vi "Results_Row_Per_Channel.vi"(0 "Duplicate Channel":bool, 1 "Duplicate Metadata channels":string[](array[string]), 2 "Analysis_info_cluster":T2={"Colour"=0, "Inst type"=enum."Pitot-static tube", "Inst name"="Manometer voltage", "Symbol"="U", "Code name"="", "Extra Info"="U", "Inst Array"=enum."PWA", "U"=0.0, "u^2"=0.0, "u^3"=0.0, "u^4"=0.0, "Skew_u"=0.0, "Kurt_u"=0.0, "Sd Error in Mean"=0.0, "% u'/U"=0.0, "X"=0.0, "Y"=0.0, "Z"=0.0, "Timescale integral Estimate"=0.0, "Sd Error in Variance"=0.0, "Calib File"=path "", "Calib Constants"=[], "Output Position"=FALSE, "Stats"=enum."None", "Av Sampling Rate"=0.0, "Av No of Samples"=0.0, "Total Meas Time (s)"=0.0, "OrigChName"="", "Max value"=0.0, "Min value"=0.0, "Req Sample Rate Hz"=0.0, "Sync Delay Time (s)"=0.0, "Ch No"=0, "Device"="", "Use Latest Calib"=FALSE, "Port"="", "Metadata Ch Names"=[], "Metadata Ch Values"=[], "Label"="", "chState"=enum."Solo", "Point Drift"=0.0, "inputConfig"=""} {"Kurt_u" format="%_3g"; "u^4" format="%_3g"; "u^3" format="%_3g"; "Sd Error in Variance" format="%_3g"; "u^2" format="%_3g"; "Sd Error in Mean" format="%_3g"; "U" format="%_3g"; "Sync Delay Time (s)" format="%.4f"; "Total Meas Time (s)" format="%_5g"; "Skew_u" format="%_3g"; "% u'/U" format="%_3g"}, 3 "Histogram Info":T1 {"X array" format="%^_5g"; "Y array" format="%^_5g"}, 4 "Index":i32) -> (5 "Channel Names":string[](array[string]), 6 "Channel Values":string[](array[string]))   [LabVIEW 2022 SP3]
uses:
  Acquisition/PWA/PWAtasksGLOBAL.vi
  Controls/Post_Process.ctl
  Globals/Meas_global.vi
  Controls/Inst_type.ctl
  FFID/FFID Calib Constants index.ctl
  Controls/Instrument_Array.ctl
  Controls/Analysis_info_cluster.ctl
  Controls/XY_Plot_Cluster.ctl
  Controls/channelState.ctl
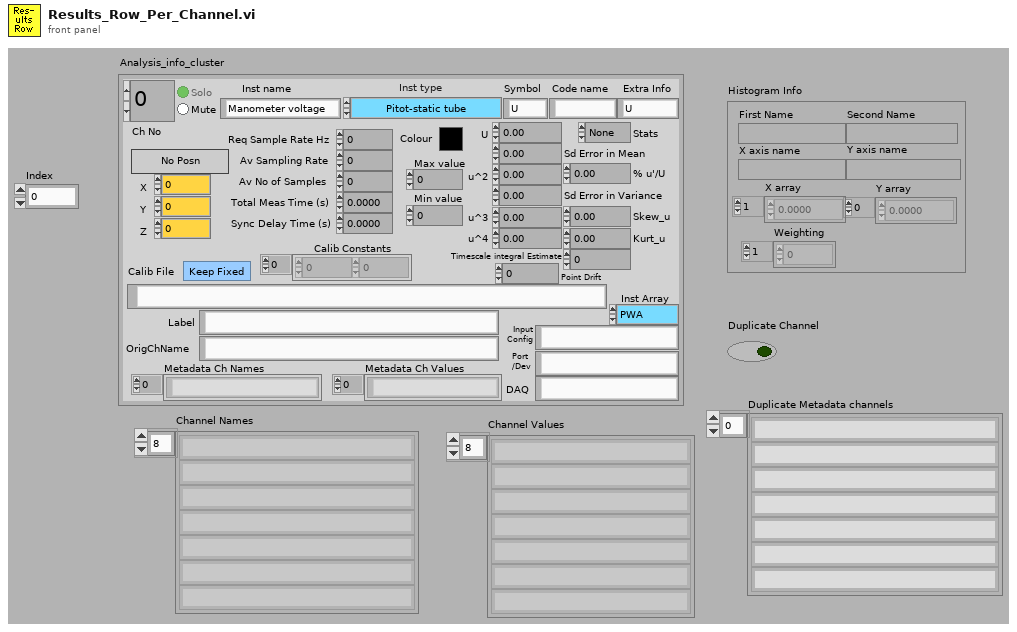
[diagram p1: front panel]
types:
  T1 = typedef "XY_Plot_Cluster.ctl" = cluster{"First Name":string, "Second Name":string, "X axis name":string, "Y axis name":string, "X array":dbl[], "Y array":dbl[], "Weighting":dbl[]}
  T2 = typedef "Analysis_info_cluster.ctl" = cluster{"Colour":u32, "Inst type":T3, "Inst name":string, "Symbol":string, "Code name":string, "Extra Info":string, "Inst Array":T4, "U":dbl, "u^2":dbl, "u^3":dbl, "u^4":dbl, "Skew_u":dbl, "Kurt_u":dbl, "Sd Error in Mean":dbl, "% u'/U":dbl, "X":dbl, "Y":dbl, "Z":dbl, "Timescale integral Estimate":dbl, "Sd Error in Variance":dbl, "Calib File":path, "Calib Constants":dbl[], "Output Position":bool, "Stats":enum16{"None", "Basic", "Full"}, "Av Sampling Rate":dbl, "Av No of Samples":dbl, "Total Meas Time (s)":dbl, "OrigChName":string, "Max value":dbl, "Min value":dbl, "Req Sample Rate Hz":dbl, "Sync Delay Time (s)":dbl, "Ch No":i16, "Device":string, "Use Latest Calib":bool, "Port":string, "Metadata Ch Names":string[], "Metadata Ch Values":string[], "Label":string, "chState":T5, "Point Drift":dbl, "inputConfig":string}
  T3 = typedef "Inst_type.ctl" = enum16{"Raw voltage", "Raw with zero offsetting", "Propeller anemometer", "Pressure Transducer", "Pitot-static tube", "Hot wire", "Cross wire 1", "Cross wire 2", "Generic Linear", "Generic Polynomial", "Generic BackPoly", "Fast FID", "Thermocouple", "Cold wire", "Pulsed Wire", "LDA Vel", "LDA Tran time", "LDA Arr time", "Microphone"}
  T4 = typedef "Instrument_Array.ctl" = enum16{"PWA", "LDA", "Analogue"}
  T5 = typedef "channelState.ctl" = enum32{"No Selection", "Solo", "Mute"}
  T6 = enum16{"Mean only", "2nd Order Stats", "4th Order Stats"}
  T7 = typedef "Post_Process.ctl" = enum16{"Take New Data", "Post Process Raw Data File"}
  T8 = typedef "FFID Calib Constants index.ctl" = u16
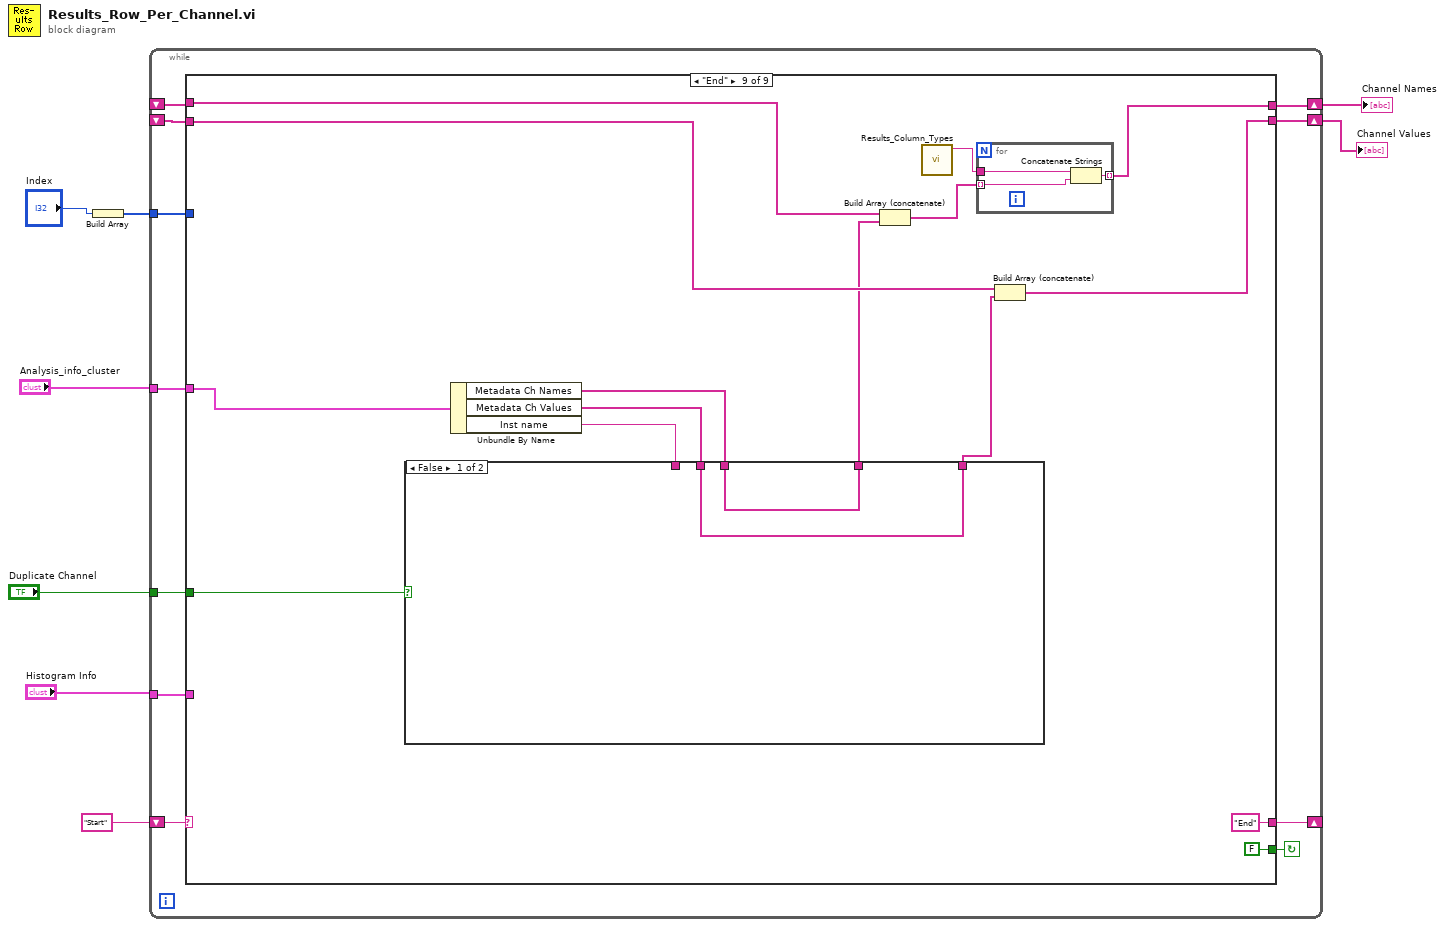
[diagram p0: block diagram]
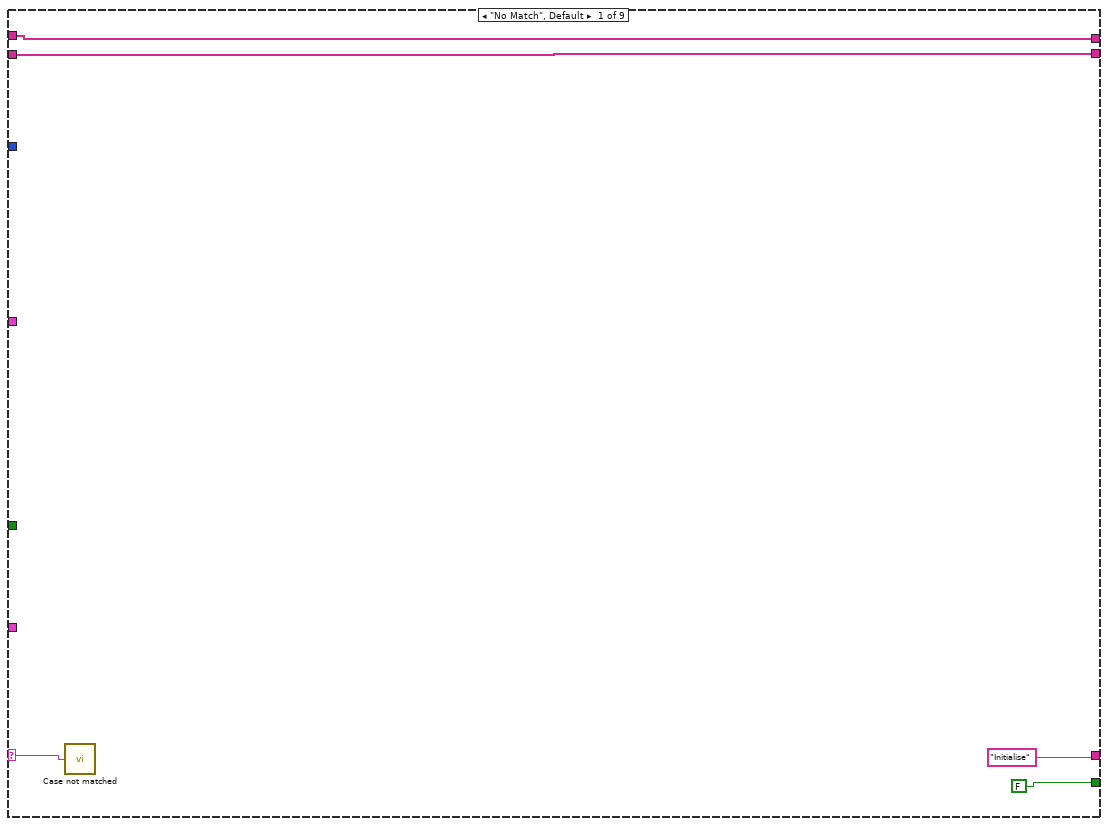
[diagram p2: hidden frame]
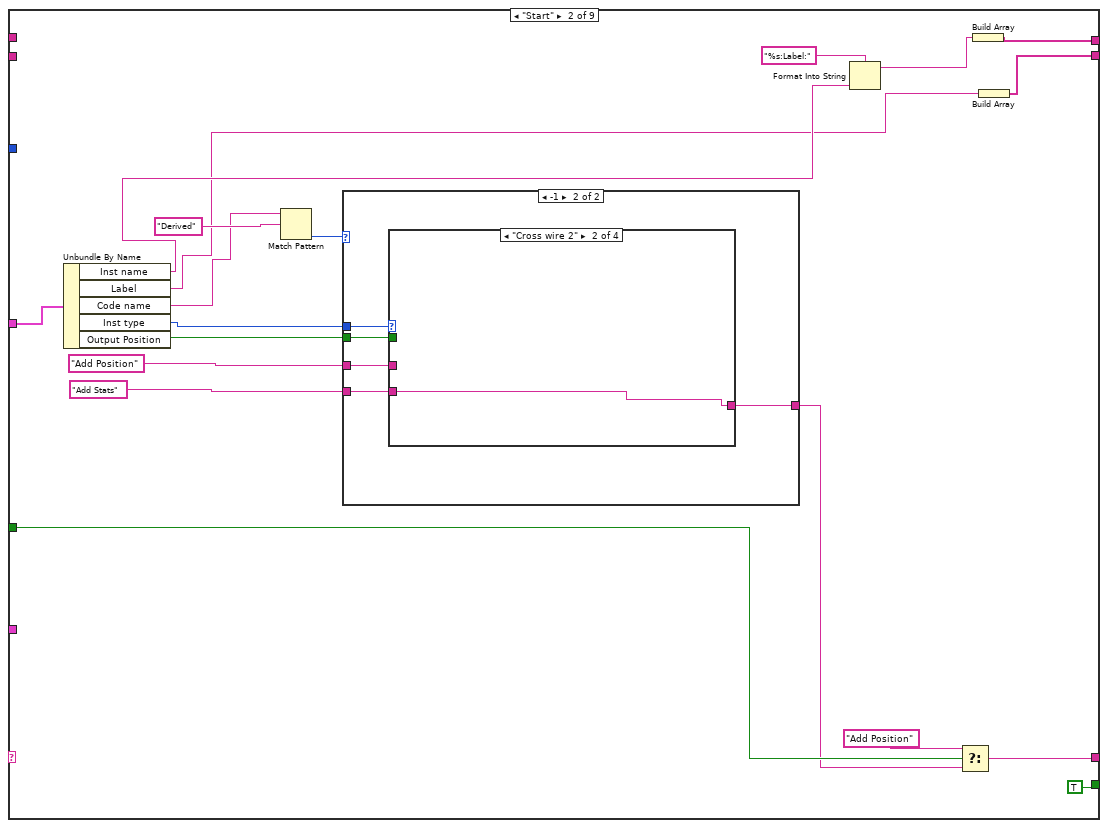
[diagram p3: hidden frame]
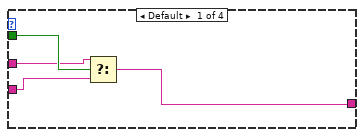
[diagram p5: hidden frame]
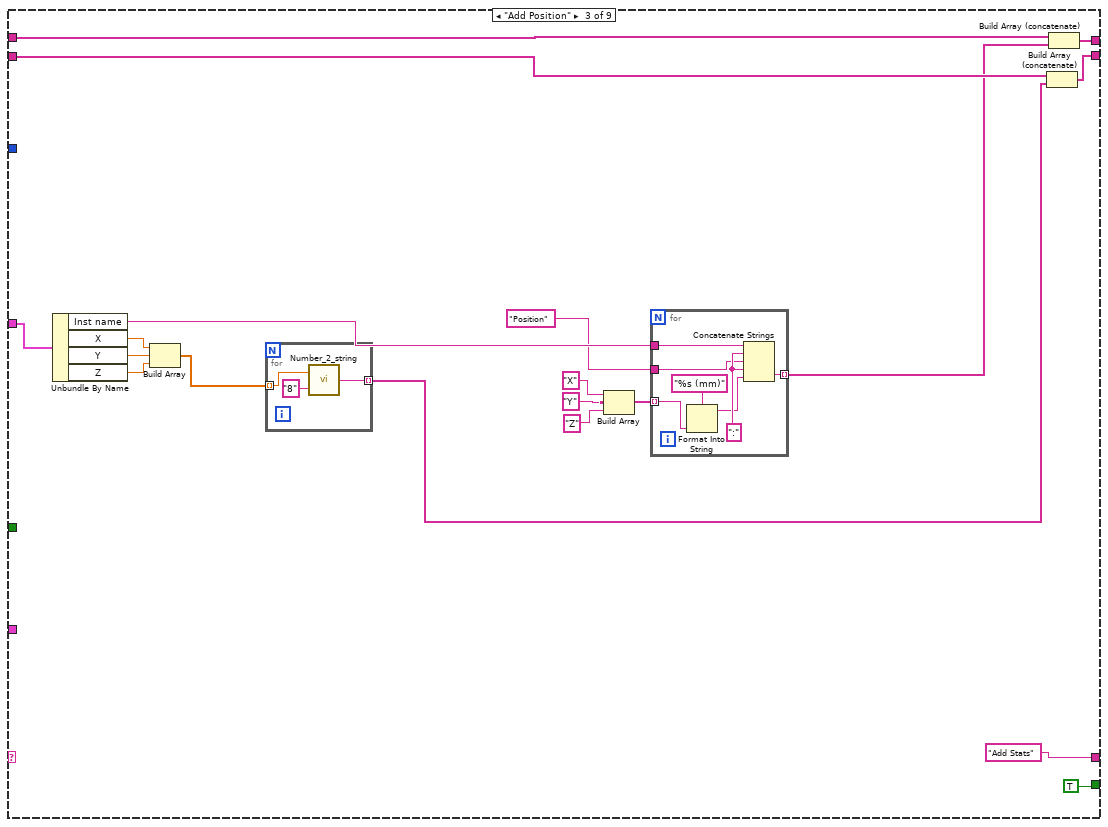
[diagram p8: hidden frame]
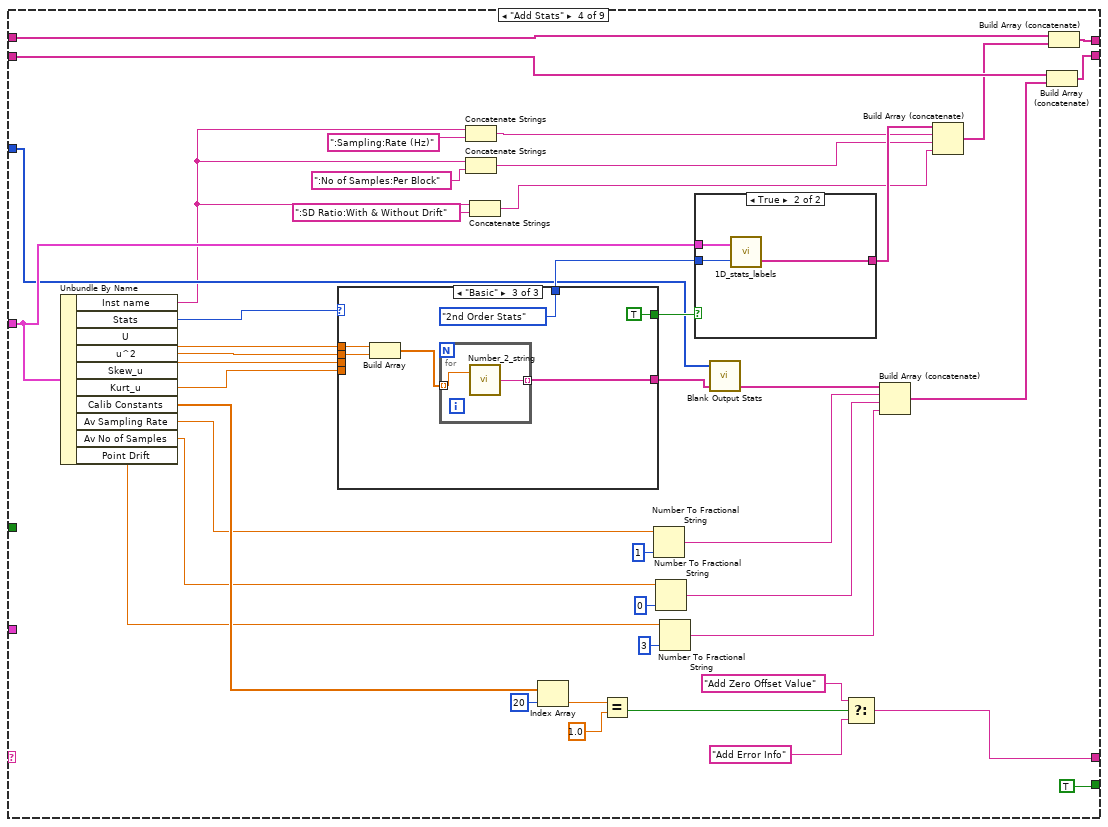
[diagram p9: hidden frame]
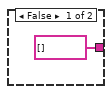
[diagram p10: hidden frame]
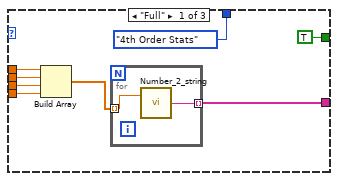
[diagram p11: hidden frame]
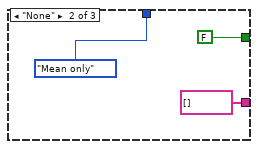
[diagram p12: hidden frame]
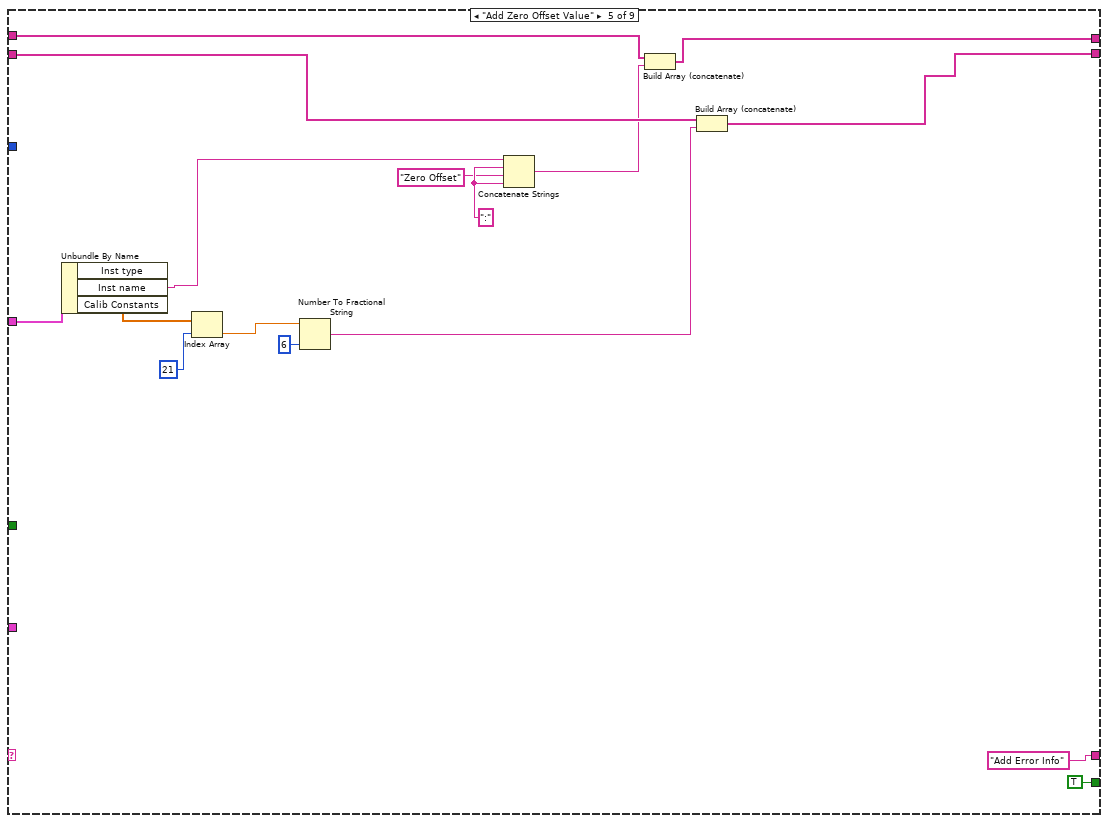
[diagram p13: hidden frame]
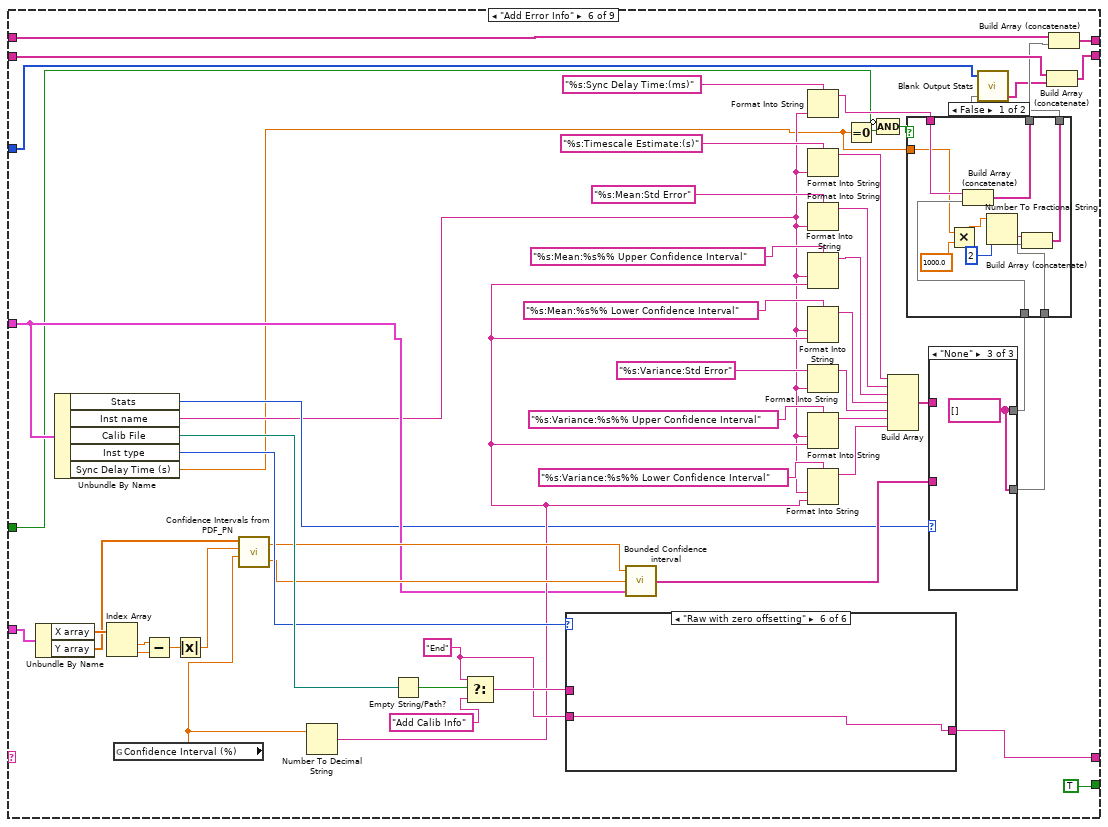
[diagram p14: hidden frame]
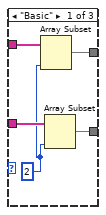
[diagram p16: hidden frame]
diagram:
  n1 = Build Array("Index") -> (w1:i32[])
  n2 = while {
    shift-left: "Start" -> [w17]
    shift-right: [w18] -> _
    shift-right: [w12] -> w5
    shift-left: _ -> [w13]
    shift-right: [w15] -> w6
    shift-left: _ -> [w14]
    tunnel: "Analysis_info_cluster" -> [w16]
    tunnel: "Histogram Info" -> [w11]
    tunnel: "Duplicate Channel" -> [w10]
    tunnel: w1 -> [w9]
    stop <- w19 continue-if-true
    n3 = case shown="\"End\"" w17 {
      selector: w17 -> [w20 _ _ _ _ _ _ _ _]
      tunnel: [FALSE TRUE TRUE TRUE TRUE TRUE TRUE TRUE FALSE] -> w19
      tunnel: ["Initialise" w31 "Add Stats" w110 "Add Error Info" w214 w255 "End" "End"] -> w18
      tunnel: w16 -> [_ w42 w73 w120 w169 w200 w268 w388 w423]
      tunnel: [w21 w25 w66 w125 w161 w222 w264 w365 w420] -> w15
      tunnel: w14 -> [w21 _ w65 w124 w163 w221 w266 w390 w421]
      tunnel: w13 -> [w22 _ w64 w123 w164 w220 w262 w389 w422]
      tunnel: [w22 w27 w63 w122 w157 w219 w260 w364 w412] -> w12
      tunnel: w11 -> [_ _ _ _ _ w211 _ _ _]
      tunnel: w10 -> [_ w34 _ _ _ w173 _ _ w415]
      tunnel: w9 -> [_ _ _ w106 _ w172 _ _ _]
      frame "No Match", Default {
        n4 = call "Case not matched.vi"("Case Name not Matched"=w20) -> ()
      }
      frame "Start" {
        n5 = Unbundle By Name(w42) -> ("Inst name"=w29:string, "Label"=w26:string, "Code name"=w37:string, "Inst type"=w41:T3, "Output Position"=w35:bool)
        n6 = Match Pattern(string=w37, regular expression="Derived") -> (offset past match=w36:i32)  [unwired: 1 in, 3 out]
        n7 = case shown="-1" w36 {
          tunnel: w41 -> [_ w49]
          tunnel: [w44 w48] -> w32
          tunnel: "Add Position" -> [_ w47]
          tunnel: "Add Stats" -> [w44 w46]
          tunnel: w35 -> [_ w45]
          frame 0, Default {
          }
          frame -1 {
            n8 = case shown="\"Cross wire 2\"" w49 {
              tunnel: [w50 w54 w55 w56] -> w48
              tunnel: w47 -> [w52 _ _ _]
              tunnel: w46 -> [w51 w54 w55 w56]
              tunnel: w45 -> [w53 _ _ _]
              frame Default {
                n9 = Select(t=w52, s=w53, f=w51) -> (s? t:f=w50:string)
              }
              frame "Cross wire 2" {
              }
              frame "LDA Tran time" {
              }
              frame "LDA Arr time" {
              }
            }
          }
        }
        n10 = Format Into String(format string="%s:Label:" ("Format String"), w29) -> (resulting string=w28:string)  [unwired: 2 in, 1 out]
        n11 = Select(t="Add Position", s=w34, f=w32) -> (s? t:f=w31:string)
        n12 = Build Array(w28) -> (w27:string[])
        n13 = Build Array(w26) -> (w25:string[])
      }
      frame "Add Position" {
        n14 = Unbundle By Name(w73) -> ("Inst name"=w72:string, "X"=w71:dbl, "Y"=w70:dbl, "Z"=w69:dbl)
        n15 = Build Array(w71, w70, w69) -> (w68:dbl[])
        n16 = for {
          tunnel: w68 -> [w78] mode=indexing
          tunnel: [w77] -> w67 mode=indexing
          n17 = call "Number_2_string.vi"("precision"="8", "number"=w78) -> ("String"=w77:string)
        }
        n18 = Build Array("X", "Y", "Z") -> (w61:string[])
        n19 = for {
          tunnel: w61 -> [w82] mode=indexing
          tunnel: w72 -> [w85]
          tunnel: [w83] -> w62 mode=indexing
          tunnel: "Position" -> [w79]
          w84 = ":" ("Substring")
          n20 = Format Into String(format string="%s (mm)", w82) -> (resulting string=w80:string)  [unwired: 2 in, 1 out]
          n21 = Concatenate Strings(w85, w84, w79, w84, w80) -> (w83:string)
        }
        n22 = Build Array (concatenate)(w65, w67) -> (w66:string[])
        n23 = Build Array (concatenate)(w64, w62) -> (w63:string[])
      }
      frame "Add Stats" {
        n24 = Unbundle By Name(w120) -> ("Inst name"=w92:string, "Stats"=w117:enum16{"None", "Basic", "Full"}, "U"=w128:dbl, "u^2"=w127:dbl, "Skew_u"=w126:dbl, "Kurt_u"=w121:dbl, "Calib Constants"=w113:dbl[], "Av Sampling Rate"=w99:dbl, "Av No of Samples"=w97:dbl, "Point Drift"=w87:dbl)
        n25 = case shown="\"Basic\"" w117 {
          tunnel: w128 -> [w140 _ w151]
          tunnel: w127 -> [w139 _ w150]
          tunnel: w126 -> [w138 _ _]
          tunnel: [w136 string[] [] w148] -> w107
          tunnel: w121 -> [w135 _ _]
          tunnel: [T6."4th Order Stats" ("Mode selector") T6."Mean only" ("Mode selector") T6."2nd Order Stats" ("Mode selector")] -> w118
          tunnel: [TRUE FALSE TRUE] -> w108
          frame "Full" {
            n26 = Build Array(w140, w139, w138, w135) -> (w137:dbl[])
            n27 = for {
              tunnel: w137 -> [w142] mode=indexing
              tunnel: [w141] -> w136 mode=indexing
              n28 = call "Number_2_string.vi"("number"=w142) -> ("String"=w141:string)  [unwired: 1 in]
            }
          }
          frame "None" {
          }
          frame "Basic" {
            n29 = Build Array(w151, w150) -> (w149:dbl[])
            n30 = for {
              tunnel: w149 -> [w153] mode=indexing
              tunnel: [w152] -> w148 mode=indexing
              n31 = call "Number_2_string.vi"("number"=w153) -> ("String"=w152:string)  [unwired: 1 in]
            }
          }
        }
        n32 = Concatenate Strings(w92, ":Sampling:Rate (Hz)" ("string")) -> (w101:string)
        n33 = Concatenate Strings(w92, ":No of Samples:Per Block") -> (w100:string)
        n34 = Concatenate Strings(w92, ":SD Ratio:With & Without Drift" ("string")) -> (w90:string)
        n35 = Index Array(array=w113, index=20) -> (element=w116:dbl)
        n36 = Equal?(x=w116, y=1.0) -> (x = y?=w112:bool)
        n37 = Number To Fractional String(number=w99, precision (6)=i16 1) -> (F-format string=w95:string)  [unwired: 2 in]
        n38 = Number To Fractional String(number=w97, precision (6)=i16 0) -> (F-format string=w94:string)  [unwired: 2 in]
        n39 = Number To Fractional String(number=w87, precision (6)=i16 3) -> (F-format string=w86:string)  [unwired: 2 in]
        n40 = case shown="True" w108 {
          tunnel: w120 -> [_ w132]
          tunnel: [string[] [] ("Output") w131] -> w102
          tunnel: w118 -> [_ w130]
          frame False {
          }
          frame True {
            n41 = call "1D_stats_labels.vi"("Mode selector"=w130, "Analysis Info Cluster"=w132) -> ("Output"=w131:string[])  [unwired: 1 in]
          }
        }
        n42 = call "Blank Output Stats.vi"("Ch Values in"=w107, "Indices"=w106) -> ("Ch Values Out"=w96:string[])  [unwired: 2 in, 1 out]
        n43 = Select(t="Add Zero Offset Value", s=w112, f="Add Error Info") -> (s? t:f=w110:string)
        n44 = Build Array (concatenate)(w96, w95, w94, w86) -> (w93:string[])
        n45 = Build Array (concatenate)(w102, w101, w100, w90) -> (w103:string[])
        n46 = Build Array (concatenate)(w124, w93) -> (w125:string[])
        n47 = Build Array (concatenate)(w123, w103) -> (w122:string[])
      }
      frame "Add Zero Offset Value" {
        w160 = ":" ("Substring")
        n48 = Unbundle By Name(w169) -> ("Inst name"=w159:string, "Calib Constants"=w168:dbl[])  [unwired: 1 out]
        n49 = Index Array(array=w168, index=21) -> (element=w165:dbl)
        n50 = Number To Fractional String(number=w165, precision (6)=i16 6) -> (F-format string=w162:string)  [unwired: 2 out]
        n51 = Concatenate Strings(w159, w160, "Zero Offset" ("string"), w160) -> (w158:string)
        n52 = Build Array (concatenate)(w164, w158) -> (w157:string[])
        n53 = Build Array (concatenate)(w163, w162) -> (w161:string[])
      }
      frame "Add Error Info" {
        w212 = "End"
        n54 = Unbundle By Name(w211) -> ("X array"=w206:dbl[], "Y array"=w205:dbl[])
        n55 = Unbundle By Name(w200) -> ("Stats"=w183:enum16{"None", "Basic", "Full"}, "Inst name"=w181:string, "Calib File"=w218:path, "Inst type"=w213:T3, "Sync Delay Time (s)"=w176:dbl)
        n56 = Index Array(array=w206) -> (element #1=w207:dbl, element #2=w208:dbl)  [unwired: 2 in]
        n57 = global read "Meas_global.vi" "Confidence Interval (%)"() -> (w202:dbl)
        n58 = Subtract(x=w207, y=w208) -> (x-y=w209:dbl)
        n59 = Absolute Value(x=w209) -> (abs(x)=w210:dbl)
        n60 = call "Confidence Intervals from PDF_PN.vi"("Desired confidence interval (%)"=w202, "PDF bin width"=w210, "Marginal 1D PDF"=w205) -> ("Lower limit scale factor on SD or SE"=w203:dbl, "Upper limit scale factor on SD or SE"=w204:dbl)  [unwired: 1 in]
        n61 = Number To Decimal String(number=w202) -> (decimal integer string=w201:string)  [unwired: 1 in]
        n62 = Empty String/Path?(string/path=w218) -> (empty?=w217:bool)
        n63 = Select(t=w212, s=w217, f="Add Calib Info") -> (s? t:f=w215:string)
        n64 = case shown="\"Raw with zero offsetting\"" w213 {
          tunnel: [w244 w245 w246 w247 w248 w249] -> w214
          tunnel: w215 -> [w244 _ _ _ _ _]
          tunnel: w212 -> [_ w245 w246 w247 w248 w249]
          frame "Propeller anemometer", Default {
          }
          frame "Cross wire 2" {
          }
          frame "LDA Tran time" {
          }
          frame "LDA Arr time" {
          }
          frame "Raw voltage" {
          }
          frame "Raw with zero offsetting" {
          }
        }
        n65 = call "Bounded Confidence interval.vi"("Analysis_info_cluster"=w200, "Lower limit scale factor on SD or SE"=w203, "Upper limit scale factor on SD or SE"=w204) -> ("Error values"=w184:string[])
        n66 = Format Into String(format string="%s:Sync Delay Time:(ms)", w181) -> (resulting string=w180:string)  [unwired: 2 in, 1 out]
        n67 = Format Into String(format string="%s:Timescale Estimate:(s)", w181) -> (resulting string=w192:string)  [unwired: 2 in, 1 out]
        n68 = Format Into String(format string="%s:Mean:Std Error", w181) -> (resulting string=w191:string)  [unwired: 2 in, 1 out]
        n69 = Format Into String(format string="%s:Mean:%s%% Upper Confidence Interval", w181, w201) -> (resulting string=w190:string)  [unwired: 2 in, 1 out]
        n70 = Format Into String(format string="%s:Mean:%s%% Lower Confidence Interval", w181, w201) -> (resulting string=w189:string)  [unwired: 2 in, 1 out]
        n71 = Format Into String(format string="%s:Variance:Std Error", w181) -> (resulting string=w188:string)  [unwired: 2 in, 1 out]
        n72 = Format Into String(format string="%s:Variance:%s%% Upper Confidence Interval", w181, w201) -> (resulting string=w187:string)  [unwired: 2 in, 1 out]
        n73 = Format Into String(format string="%s:Variance:%s%% Lower Confidence Interval", w181, w201) -> (resulting string=w186:string)  [unwired: 2 in, 1 out]
        n74 = Equal To 0?(x=w176) -> (x = 0?=w175:bool)
        n75 = Compound Arithmetic op=AND(invert w173, w175) -> (w174:bool)
        n76 = Build Array(w192, w191, w190, w189, w188, w187, w186) -> (w185:string[])
        n77 = case shown="\"None\"" w183 {
          tunnel: w185 -> [w240 w242 _]
          tunnel: [w239 w242 w243] -> w179
          tunnel: w184 -> [w238 w241 _]
          tunnel: [w237 w241 w243] -> w177
          frame "Basic" {
            w236 = 2 ("length")
            n78 = Array Subset(array=w240, length=w236) -> (w239:string[])  [unwired: 1 in]
            n79 = Array Subset(array=w238, length=w236) -> (w237:string[])  [unwired: 1 in]
          }
          frame "Full" {
          }
          frame "None" {
            w243 = string[] []
          }
        }
        n80 = case shown="False" w174 {
          tunnel: w180 -> [w233 _]
          tunnel: w179 -> [w232 w235]
          tunnel: [w231 w235] -> w178
          tunnel: w177 -> [w230 w234]
          tunnel: [w229 w234] -> w171
          tunnel: w176 -> [w228 _]
          frame False {
            n81 = Multiply(x=w228, y=1000.0) -> (x*y=w226:dbl)
            n82 = Build Array (concatenate)(w233, w232) -> (w231:string[])
            n83 = Number To Fractional String(number=w226, precision (6)=i16 2) -> (F-format string=w225:string)  [unwired: 2 in]
            n84 = Build Array (concatenate)(w225, w230) -> (w229:string[])
          }
          frame True {
          }
        }
        n85 = call "Blank Output Stats.vi"("Ch Values in"=w171, "Indices"=w172) -> ("Ch Values Out"=w170:string[])  [unwired: 2 in, 1 out]
        n86 = Build Array (concatenate)(w221, w170) -> (w222:string[])
        n87 = Build Array (concatenate)(w220, w178) -> (w219:string[])
      }
      frame "Add Calib Info" {
        w250 = T8 19 items=["0 Coeff A", "1 Coeff B", "2 Coeff C", "3 FFID Bkgnd", "4 FFID Bkgnd Variance", "5 FFID Bkgnd Volts", "6 FFID Bkgnd Time", "7 GMU Source ppm/%density", "8 Orig Bkgnd Time", "9 Orig Bknd volts", "10 Orig bkgnd Variance", "11 Intermittency Theshold", "12 Intermittency", "13 Head Temp", "14 Exhaust Temp", "15", "16", "17", "18 Calibration Drift %", "19 Calibration Interval Minutes"] ("FFID")
        w251 = T8 18 items=["0 Coeff A", "1 Coeff B", "2 Coeff C", "3 FFID Bkgnd", "4 FFID Bkgnd Variance", "5 FFID Bkgnd Volts", "6 FFID Bkgnd Time", "7 GMU Source ppm/%density", "8 Orig Bkgnd Time", "9 Orig Bknd volts", "10 Orig bkgnd Variance", "11 Intermittency Theshold", "12 Intermittency", "13 Head Temp", "14 Exhaust Temp", "15", "16", "17", "18 Calibration Drift %", "19 Calibration Interval Minutes"] ("FFID")
        n88 = Unbundle By Name(w268) -> ("Inst name"=w259:string, "Inst type"=w258:T3, "Calib Constants"=w252:dbl[], "Calib File"=w267:path)
        n89 = Format Into String(format string="%s:Calibration:Filename" ("Format String"), w259) -> (resulting string=w261:string)  [unwired: 2 in, 1 out]
        n90 = Strip Path(path=w267) -> (name=w265:string)  [unwired: 1 out]
        n91 = case shown="\"Generic Linear\", Default" w258 {
          tunnel: [w275 w280 w297 w303 w310 w333] -> w264
          tunnel: w266 -> [w273 w281 w298 w304 w311 w334]
          tunnel: w265 -> [w274 w279 w296 w302 _ w327]
          tunnel: w252 -> [_ _ w289 _ _ w326]
          tunnel: w262 -> [w272 w278 w295 w301 w307 w321]
          tunnel: w261 -> [w270 w277 w294 w299 w305 w320]
          tunnel: [w271 w276 w293 w300 w306 w315] -> w260
          tunnel: w259 -> [_ _ w291 _ _ w314]
          tunnel: w250 -> [_ _ _ _ _ w313]
          tunnel: w251 -> [_ _ _ _ _ w312]
          frame "Propeller anemometer" {
            n92 = Build Array (concatenate)(w272, w270) -> (w271:string[])
            n93 = Build Array (concatenate)(w273, w274) -> (w275:string[])
          }
          frame "Pressure Transducer" {
            n94 = Build Array (concatenate)(w278, w277) -> (w276:string[])
            n95 = Build Array (concatenate)(w281, w279) -> (w280:string[])
          }
          frame "Cold wire" {
            n96 = Index Array(array=w289, index #1=7 ("index"), index #2=6 ("index")) -> (element #1=w283:dbl, element #2=w282:dbl)
            n97 = Format Into String(format string="%s:Mean:Voltage" ("Format String"), w291) -> (resulting string=w290:string)  [unwired: 2 in, 1 out]
            n98 = Divide(x=w283, y=w282) -> (x/y=w287:dbl)
            n99 = Number To Fractional String(number=w287, precision (6)=i16 6) -> (F-format string=w285:string)  [unwired: 2 in]
            n100 = Build Array (concatenate)(w295, w294, w290) -> (w293:string[])
            n101 = Build Array (concatenate)(w298, w296, w285) -> (w297:string[])
          }
          frame "Pitot-static tube" {
            n102 = Build Array (concatenate)(w301, w299) -> (w300:string[])
            n103 = Build Array (concatenate)(w304, w302) -> (w303:string[])
          }
          frame "Pulsed Wire" {
            n104 = global read "PWAtasksGLOBAL.vi" "PWA Calib. File Path"() -> (w309:path)
            n105 = Strip Path(path=w309) -> (name=w308:string)  [unwired: 1 out]
            n106 = Build Array (concatenate)(w307, w305) -> (w306:string[])
            n107 = Build Array (concatenate)(w311, w308) -> (w310:string[])
          }
          frame "Generic Linear", Default {
            n108 = global read "Meas_global.vi" "Post Process"() -> (w329:T7)
            n109 = Index Array(array=w326, index=w312) -> (element=w332:dbl)
            n110 = Format Into String(format string="%s:Calibration:Drift:%%" ("Format String"), w314) -> (resulting string=w317:string)  [unwired: 2 in, 1 out]
            n111 = Not A Number/Path/Refnum?(number/path/refnum=w332) -> (NaN/Path/Refnum?=w331:bool)
            n112 = Equal?(x=w329, y=Post_Process."Post Process Raw Data File" ("Post Process")) -> (x = y?=w322:bool)
            n113 = case shown="False" w331 {
              tunnel: [w344 w349] -> w328
              tunnel: w332 -> [w345 _]
              tunnel: w322 -> [_ w351]
              tunnel: w327 -> [_ w348]
              frame False {
                n114 = Number To Fractional String(number=w345, precision (6)=i16 2) -> (F-format string=w344:string)  [unwired: 2 out]
              }
              frame True {
                n115 = Concatenate Strings(w348, "_Drift_Place_Holder" ("Substring")) -> (w350:string)
                n116 = Select(t="No Info", s=w351, f=w350) -> (s? t:f=w349:string)
              }
            }
            n117 = Index Array(array=w326, index=w313) -> (element=w325:dbl)
            n118 = Not A Number/Path/Refnum?(number/path/refnum=w325) -> (NaN/Path/Refnum?=w324:bool)
            n119 = case shown="False" w324 {
              tunnel: [w335 w340] -> w323
              tunnel: w325 -> [w336 _]
              tunnel: w322 -> [_ w342]
              tunnel: w327 -> [_ w339]
              frame False {
                n120 = Number To Fractional String(number=w336, precision (6)=i16 2) -> (F-format string=w335:string)  [unwired: 2 out]
              }
              frame True {
                n121 = Concatenate Strings(w339, "_Interval_Place_Holder" ("Substring")) -> (w341:string)
                n122 = Select(t="No Info", s=w342, f=w341) -> (s? t:f=w340:string)
              }
            }
            n123 = Format Into String(format string="%s:Calibration:Interval:Minutes" ("Format String"), w314) -> (resulting string=w316:string)  [unwired: 2 in, 1 out]
            n124 = Build Array (concatenate)(w334, w327, w328, w323) -> (w333:string[])
            n125 = Build Array (concatenate)(w321, w320, w317, w316) -> (w315:string[])
          }
        }
        n126 = Equal?(x=w258, y=Inst_type."Fast FID" ("Inst type")) -> (x = y?=w257:bool)
        n127 = Select(t="Add FFID Info", s=w257, f="End") -> (s? t:f=w255:string)
      }
      frame "Add FFID Info" {
        w353 = T8[] [12, 3, 4, 11, 7, 8, 9, 10, 13, 14] items=["0 Coeff A", "1 Coeff B", "2 Coeff C", "3 FFID Bkgnd", "4 FFID Bkgnd Variance", "5 FFID Bkgnd Volts", "6 FFID Bkgnd Time", "7 GMU Source ppm/%density", "8 Orig Bkgnd Time", "9 Orig Bknd volts", "10 Orig bkgnd Variance", "11 Intermittency Theshold", "12 Intermittency", "13 Head Temp", "14 Exhaust Temp", "15", "16", "17", "18 Calibration Drift %", "19 Calibration Interval Minutes"] ("Calib Constants")
        n128 = Unbundle By Name(w388) -> ("U"=w375:dbl, "Inst name"=w386:string, "Calib Constants"=w376:dbl[])
        n129 = Index Array(array=w376, index=3) -> (element=w379:dbl)
        n130 = Array Subset(array=w376, length=3) -> (w368:dbl[])  [unwired: 1 in]
        n131 = for {
          tunnel: w376 -> [w410]
          tunnel: w353 -> [w409] mode=indexing
          tunnel: [w406] -> w359 mode=indexing
          tunnel: string[] ["", "", "", "", "", "", "7", "", " ", " "] -> [w407] mode=indexing
          tunnel: [w406] -> w362
          n132 = Index Array(array=w410, index=w409) -> (element=w408:dbl)
          n133 = call "Number_2_string.vi"("precision"=w407, "number"=w408) -> ("String"=w406:string)
        }
        n134 = Add(x=w375, y=w379) -> (x+y=w374:dbl)
        n135 = Index Array(array=w376, index=3) -> (element=w372:dbl)
        n136 = call "Polybackwards.vi"("Coefficients"=w368, "Y input"=w374) -> ("X output"=w383:dbl)  [unwired: 1 out]
        n137 = call "Polybackwards.vi"("Coefficients"=w368, "Y input"=200.0) -> ("X output"=w369:dbl)  [unwired: 1 out]
        n138 = call "Polybackwards.vi"("Coefficients"=w368, "Y input"=w372) -> ("X output"=w371:dbl)  [unwired: 1 out]
        n139 = call "Number_2_string.vi"("precision"="5", "number"=w369) -> ("String"=w366:string)
        n140 = call "Number_2_string.vi"("precision"="5", "number"=w383) -> ("String"=w381:string)
        n141 = call "Number_2_string.vi"("precision"="5", "number"=w371) -> ("String"=w373:string)
        n142 = Equal?(x=w362, y="0") -> (x = y?=w361:bool)
        n143 = for {
          tunnel: string[] ["Measured", "Bkgnd", "Voltage for 200ppm", "Intermittency", "Bkgnd", "Bkgnd Variance", "Threshold", "Calibration", "Orig Bkgnd Time", "Orig Bkgnd", "Orig Bkgnd Variance", "Head Temp", "Exhaust Temp"] ("appended array") -> [w402] mode=indexing
          tunnel: w386 -> [w403]
          tunnel: [w404] -> w360 mode=indexing
          tunnel: string[] ["Volts", "Volts", "Volts", "", "ppm", "ppm^2", "ppm", "ppm/%Density", "Sec", "Volts", "ppm^2", "deg C", "deg C"] ("appended array") -> [w401] mode=indexing
          w405 = ":" ("Substring")
          n144 = Concatenate Strings(w403, w405, w402, w405, w401) -> (w404:string)
        }
        n145 = case shown="True" w361 {
          tunnel: [w393 w399] -> w356
          tunnel: w360 -> [w393 w400]
          tunnel: [w392 w397] -> w357
          tunnel: w359 -> [w392 w398]
          tunnel: 8 -> [_ w396]
          frame False {
          }
          frame True {
            n146 = Add(x=w396, y=3) -> (x+y=w394:i32)
            n147 = Array Subset(array=w398, length=w396) -> (w397:string[])  [unwired: 1 in]
            n148 = Array Subset(array=w400, length=w394) -> (w399:string[])  [unwired: 1 in]
          }
        }
        n149 = Build Array (concatenate)(w389, w356) -> (w364:string[])
        n150 = Build Array (concatenate)(w390, w381, w373, w366, w357) -> (w365:string[])
      }
      frame "End" {
        n151 = Unbundle By Name(w423) -> ("Metadata Ch Names"=w419:string[], "Metadata Ch Values"=w416:string[], "Inst name"=w414:string)
        n152 = case shown="False" w415 {
          tunnel: w414 -> [_ w436]
          tunnel: w419 -> [w430 w434]
          tunnel: [w430 w433] -> w418
          tunnel: [w429 w432] -> w417
          tunnel: w416 -> [w429 w431]
          frame False {
          }
          frame True {
            n153 = for {
              tunnel: w436 -> [w444]
              tunnel: "Duplicate Metadata channels" -> [w438] mode=indexing
              tunnel: w434 -> [w443]
              tunnel: [w441] -> w433 mode=indexing
              tunnel: [w440] -> w432 mode=indexing
              tunnel: w431 -> [w439]
              n154 = Concatenate Strings(w444, ":" ("string"), w438) -> (w441:string)
              n155 = Search 1D Array(1D array=w443, element=w441) -> (index of element=w442:i32)  [unwired: 1 in]
              n156 = case shown="-1" w442 {
                selector: w442 -> [w446 _]
                tunnel: [w445 ""] -> w440
                tunnel: w439 -> [w447 _]
                frame Default {
                  n157 = Index Array(array=w447, index=w446) -> (element=w445:string)
                }
                frame -1 {
                }
              }
            }
          }
        }
        n158 = Build Array (concatenate)(w422, w418) -> (w413:string[])
        n159 = call "Results_Column_Types.vi"() -> ("Instrument"=w411:string)  [unwired: 9 in, 2 out]
        n160 = for {
          tunnel: w413 -> [w428] mode=indexing
          tunnel: [w427] -> w412 mode=indexing
          tunnel: w411 -> [w426]
          n161 = Concatenate Strings(w426, w428) -> (w427:string)
        }
        n162 = Build Array (concatenate)(w421, w417) -> (w420:string[])
      }
    }
  }
  "Channel Names" <- w5
  "Channel Values" <- w6
